vi "create bit sequence.vi"(8 "error in (no error)":errorcluster, 9 "Enum":enum16{"Pseudo-random sequence", "Text"}(ring), 10 "total bits (128)":i32, 11 "String":string) -> (0 "error out":errorcluster, 3 "output bit stream":i8[](array[numeric]))   [LabVIEW 2022 SP3]
uses:
  <vilib>/addons/Modulation/Digital/General/MT Generate Bits (Galois, PN Order).vi
  <vilib>/addons/Modulation/Digital/Support/Common/Validators/mod_Generate Bits Validate.vi
  <vilib>/addons/Modulation/Analog/support/mod_Set Error Source.vi
  <vilib>/addons/Modulation/Digital/General/subVIs/mod_Generate Bits PN Sequence.vi
  <vilib>/addons/Modulation/Digital/General/MT Generate Bits (User Defined).vi
  <vilib>/addons/Modulation/niDMT.lvlib
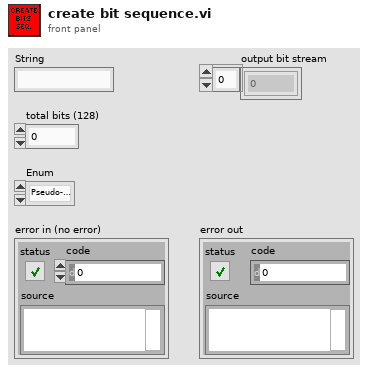
[diagram p1: front panel]
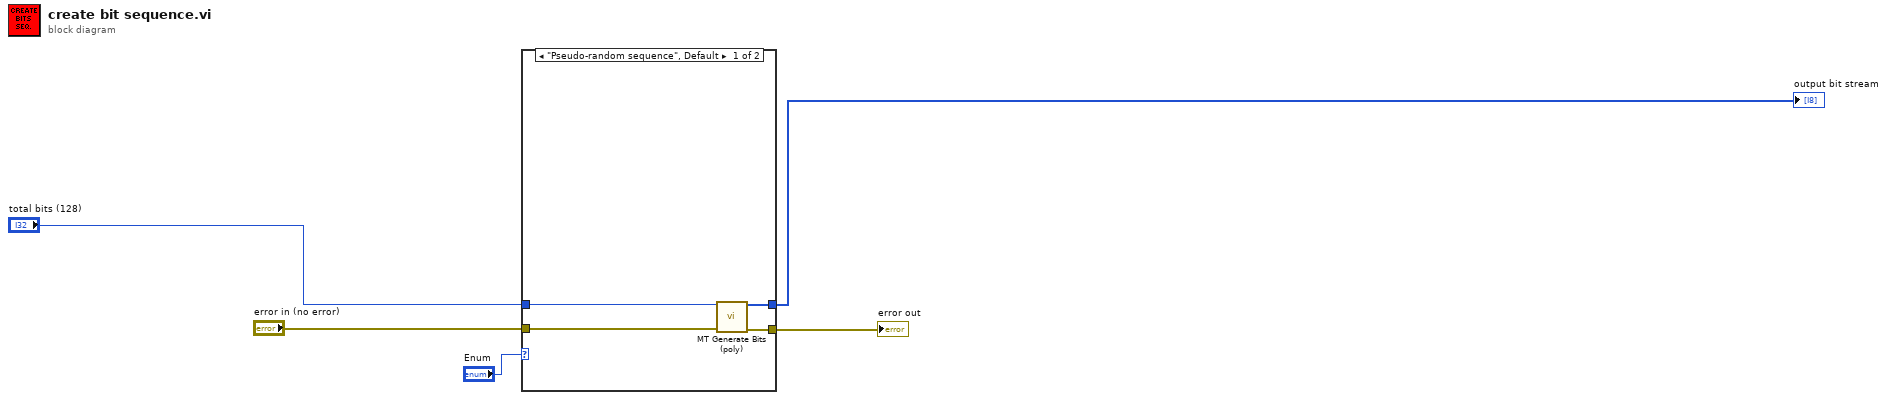
[diagram p0: block diagram]
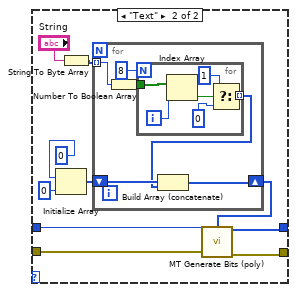
[diagram p2: hidden frame]
diagram:
  n1 = case shown="\"Pseudo-random sequence\", Default" "Enum" {
    tunnel: "total bits (128)" -> [w9 w19]
    tunnel: [w8 w10] -> w2
    tunnel: "error in (no error)" -> [w7 w11]
    tunnel: [w6 w14] -> w4
    frame "Pseudo-random sequence", Default {
      n2 = call-poly <vilib>:"MT Generate Bits (poly).vi"("total bits (128)"=w9, "error in (no error)"=w7) -> ("output bit stream"=w6:i8[], "error out"=w8:errorcluster)  [unwired: 11 in, 1 out]
    }
    frame "Text" {
      n3 = Initialize Array(i8 0, 0 ("dimension size")) -> (w15:i8[])
      n4 = String To Byte Array(string="String") -> (unsigned byte array=w18:u8[])
      n5 = for {
        tunnel: w18 -> [w24] mode=indexing
        shift-right: [w20] -> w13
        shift-left: w15 -> [w22]
        n6 = Number To Boolean Array(number=w24) -> (Boolean array=w23:bool[])
        n7 = for {
          N: 8 -> [_]
          tunnel: w23 -> [w30]
          tunnel: [w26] -> w21 mode=indexing
          i -> [w31]
          n8 = Index Array(array=w30, index=w31) -> (element=w29:bool)
          n9 = Select(t=i8 1, s=w29, f=i8 0) -> (s? t:f=w26:i8)
        }
        n10 = Build Array (concatenate)(w22, w21) -> (w20:i8[])
      }
      n11 = call-poly <vilib>:"MT Generate Bits (poly).vi"("total bits (128)"=w19, "user base bit pattern"=w13, "error in (no error)"=w11) -> ("output bit stream"=w14:i8[], "error out"=w10:errorcluster)  [unwired: 11 in]
    }
  }
  "output bit stream" <- w4
  "error out" <- w2
